vi "Actor Core.vi"(8 "error in":errorcluster, 11 "Chat Window Model in":refnum<class "Chat Window Model.lvclass">) -> (0 "error out":errorcluster, 3 "Actor out":refnum<class "Actor.lvclass">)   [LabVIEW 2015, in "Chat Window Model.lvlib" / "Chat Window Model.lvclass"]
doc: "(<B>Filename</B>: Actor Framework.lvlib:Actor.lvclass:Actor Core.vi)\n\nReceives messages to the actor, reacts to them, and initiates any error handling that may shut the actor down.\n\nDescendant classes may override this VI to append parallel tasks for the actor to complete while it handles messages. Overrides use the Call Parent Method node."
uses:
  Chat Window Model.lvclass
  <vilib>/ActorFramework/Actor/Actor.lvclass
  Chat Window Interface/Chat Window Interface.lvclass
  Chat Window Model Messages/User Updated Status Msg/User Updated Status Msg.lvclass
  Chat Window Model Messages/Forward Direct Message Msg/Forward Direct Message Msg.lvclass
  Chat Window Model Messages/New Panel Launched Msg/New Panel Launched Msg.lvclass
  Chat Window UI Controller/Chat Window UI Controller/Chat Window UI Controller.lvclass/Chat Window UI Controller.ctl
  Chat Window Model.lvclass/Chat Window Model.ctl
  Chat Window UI Controller/Chat Window UI Controller/Chat Window UI Controller.lvclass
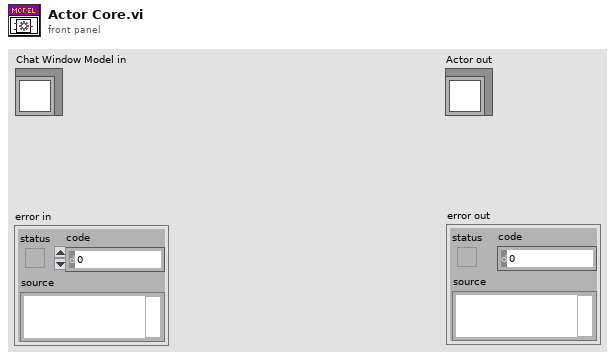
[diagram p1: front panel]
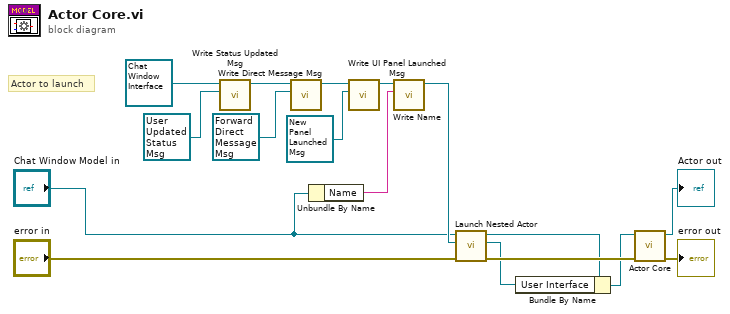
[diagram p0: block diagram]
diagram:
  # "Actor to launch"
  n1 = call "Write Status Updated Msg.vi"("Chat Window UI Controller.lvlib:Status Updated Msg.lvclass"=refnum<class "User Updated Status Msg.lvclass"> refnum ("Chat Window Model.lvlib:User Updated Status Msg.lvclass"), "Chat Window UI Controller in"=refnum<class "Chat Window Interface.lvclass"> refnum ("Chat Window Interface.lvlib:Chat Window Interface.lvclass")) -> ("Chat Window UI Controller out"=w8:refnum<class "Chat Window Interface.lvclass">)  [unwired: 9 in]
  n2 = call "Write Direct Message Msg.vi"("Chat Window UI Controller.lvlib:Direct Message Msg.lvclass"=refnum<class "Forward Direct Message Msg.lvclass"> refnum ("Chat Window Model.lvlib:Forward Direct Message Msg.lvclass"), "Chat Window UI Controller in"=w8) -> ("Chat Window UI Controller out"=w2:refnum<class "Chat Window Interface.lvclass">)  [unwired: 9 in]
  n3 = Unbundle By Name("Chat Window Model in") -> ("Name"=w4:string)
  n4 = call "Write UI Panel Launched Msg.vi"("Chat Window UI Controller.lvlib:UI Panel Launched Msg.lvclass"=refnum<class "New Panel Launched Msg.lvclass"> refnum ("Chat Window Model.lvlib:New Panel Launched Msg.lvclass"), "Chat Window UI Controller in"=w2) -> ("Chat Window UI Controller out"=w3:refnum<class "Chat Window Interface.lvclass">)  [unwired: 9 in]
  n5 = call "Write Name.vi"("Name"=w4, "Chat Window UI Controller in"=w3) -> ("Chat Window UI Controller out"=w6:refnum<class "Chat Window Interface.lvclass">)  [unwired: 8 in, 1 out]
  n6 = call <vilib>:"Launch Nested Actor.vi"("error in (no error)"="error in", "Nested Actor"=w6, "Caller Actor in"="Chat Window Model in") -> ("error out"=w14:errorcluster, "Nested Actor's Enqueuer"=w11:refnum<class "Message Enqueuer.lvclass">, "Caller Actor out"=w12:refnum<class "Chat Window Model.lvclass">)  [unwired: 6 in]
  n7 = Bundle By Name(cluster=w12, "User Interface"=w11) -> (w13:refnum<class "Chat Window Model.lvclass">)
  n8 = call-parent "Actor Core.vi"("error in"=w14, "Actor in"=w13) -> ("error out"=→"error out":errorcluster, "Actor out"=→"Actor out":refnum<class "Actor.lvclass">)  [unwired: 8 in]
